vi "LVClass_WavefrontCorrector Set Parameter Real.vi"(0 "WavefrontCorrector in":refnum<class "WavefrontCorrector.lvclass">, 5 "parameter_name":string, 9 "value":sgl, 11 "error in (no error)":errorcluster) -> (4 "WavefrontCorrector out":refnum<class "WavefrontCorrector.lvclass">, 15 "error out":errorcluster)   [LabVIEW 2020, in "WavefrontCorrector.lvclass"]
doc: "WavefrontCorrector parameter setter for parameter of type float.\n\n--------------------------------------------------------------------------------\n\n<B>correctorIn </B> : WavefrontCorrector object.\n<B>correctorOut </B> : WavefrontCorrector object.\n<B>parameter_name </B> : Name of the parameter.\n<B>value </B> : Value of the parameter.\n<B>ErrorIn </B> : Error\n<B>ErrorOut </B> : Error\n\n--------------------------------------------------------------------------------"
uses:
  WavefrontCorrector.lvclass
  WavefrontCorrector.lvclass/WavefrontCorrector.ctl
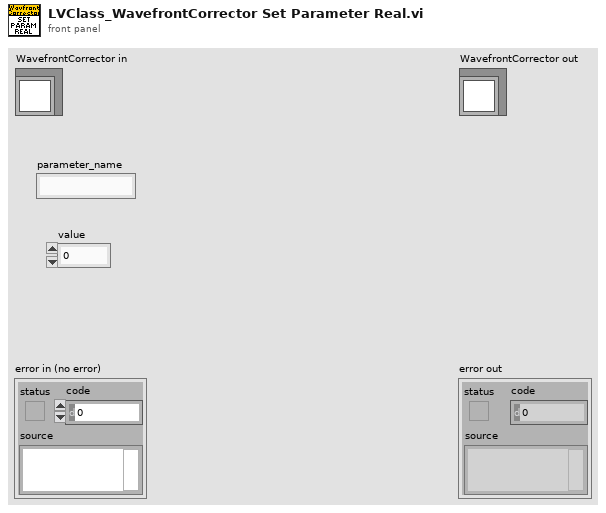
[diagram p1: front panel]
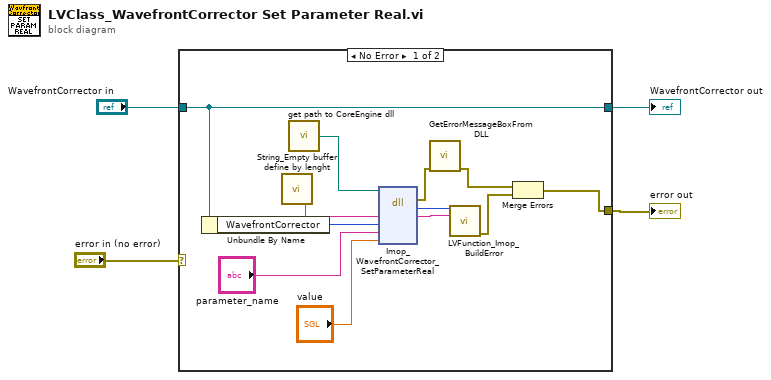
[diagram p0: block diagram]
diagram:
  n1 = case shown="No Error" "error in (no error)" {
    selector: "error in (no error)" -> [_ w18]
    tunnel: [w5 w18] -> w2
    tunnel: [w12 w17] -> w1
    tunnel: "WavefrontCorrector in" -> [w12 w17]
    frame No Error {
      n2 = Unbundle By Name(w12) -> ("WavefrontCorrector"=w13:i32)
      n3 = call "String_Empty buffer define by lenght.vi"() -> ("Empty buffer"=w16:string)  [unwired: 1 in]
      n4 = call "get path to CoreEngine dll.vi"() -> ("path to c_interface_vc100.dll"=w11:path)  [unwired: 12 in, 3 out]
      n5 = dll-call lib="D:/soft/HASO_v3/SVN_trunk/ImOpCoreEngine4_LV2011/DLLs/c_interface_vc100.dll" fn="Imop_WavefrontCorrector_SetParameterReal"(path in=w11, "message"=w16, "camera"=w13, "parameter_name"="parameter_name", "value"="value") -> (error out=w10:errorcluster, "return type"=w15:i32, "message"=w14:string)  [unwired: 5 in, 1 out]
      n6 = call "GetErrorMessageBoxFromDLL.vi"("error IN"=w10) -> ("error OUT"=w7:errorcluster)  [unwired: 10 in]
      n7 = call "LVFunction_Imop_BuildError.vi"("code"=w15, "String to Prepend to source (\"\")"=w14) -> ("error out"=w6:errorcluster)  [unwired: 13 in]
      n8 = Merge Errors(w7, w6) -> (w5:errorcluster)
    }
    frame Error {
    }
  }
  "error out" <- w2
  "WavefrontCorrector out" <- w1
